vi "Drive_Cmd_Follow_Camera.vi"(9 "Forward Power":dbl, 10 "Max Turn Power":dbl, 11 "Drive Loop Cluster":T1={"Sensor Data"={"Gyro Data"={"Gyro RT FIFO"=refnum, "Gyro Current"=0.0, "Gyro Hold"=0.0}, "Encoder Data"={"Encoder RT FIFO"=refnum, "Encoder Current"=0.0, "Encoder Hold"=0.0}, "Camera Data"={"Camera RT FIFO"=refnum, "Camera Current"={" Angle"=0.0, "Valid"=FALSE}}}, "PID Update"=refnum, "RobotDriveDevRef"={"DevStatus"={"status"=FALSE, "code"=0, "source"=""}, "Motors[]"=[], "Square Inputs"=FALSE, "Max Output"=1.0}, "Drive Train"=enum."Tank Drive 2 Motor", "Valid Commands"=[], "Drive Comand Notifier"=refnum, "Command Finished?"=refnum, "Command Canceled"=refnum}) -> (0 "error out":errorcluster)   [LabVIEW 2016]
doc: "Help file written by FRC Team 836 - The RoboBees\n\nThis VI writes the \"Follow Camera\" command and power level #6 to the Drive Command RT FIFO in the Drive Loop Cluster.\n\nThe RT FIFO has to be initialized using the \"Drive_Loop_Initialize_w_Help\" VI"
uses:
  <userlib>/836-libraries/Drive/Drive_Code_V2/Drive_Code_Support/Drive_Code_Bundle.ctl
  <userlib>/836-libraries/Drive/Drive_Code_V2/Drive_Code_Support/SensorTypedefs/Sensor_Cluster.ctl
  <userlib>/836-libraries/Drive/Drive_Code_V2/Drive_Code_Support/SensorTypedefs/Camera_Cluster.ctl
  <userlib>/836-libraries/Drive/Drive_Code_V2/Drive_Code_Support/PidClusters/Drive_Code_PID_Bundle.ctl
  <vilib>/Rock Robotics/WPI/RobotDrive/WPI_RobotDriveDevRef.ctl
  <vilib>/Rock Robotics/WPI/MotorControl/WPI_MotorControlDeviceRef.ctl
  <vilib>/Rock Robotics/WPI/MotorControl/WPI_MotorControlType.ctl
  <vilib>/Rock Robotics/SystemInterfaces/DIO/FPGA_DIOPWMChannel.ctl
  <vilib>/Rock Robotics/WPI/PWM/WPI_PWMDeadband.ctl
  <userlib>/836-libraries/Drive/Drive_Code_V2/Drive_Code_Support/DriveTrains/Drive_Trains.ctl
  <userlib>/836-libraries/Drive/Drive_Code_V2/Drive_Code_Support/Command_Sends/Drive_Code_Command_Type.ctl
  <userlib>/836-libraries/Drive/Drive_Code_V2/Drive_Code_Support/Command_Sends/Drive_Code_Command_List.ctl
  <userlib>/836-libraries/Drive/Drive_Code_V2/Drive_Code_Support/Command_Sends/CommandTypeInfo/FollowCameraparam.ctl
  <vilib>/Utility/error.llb/Error Cluster From Error Code.vi
  <vilib>/ErrorRing/Error Ring.xnode
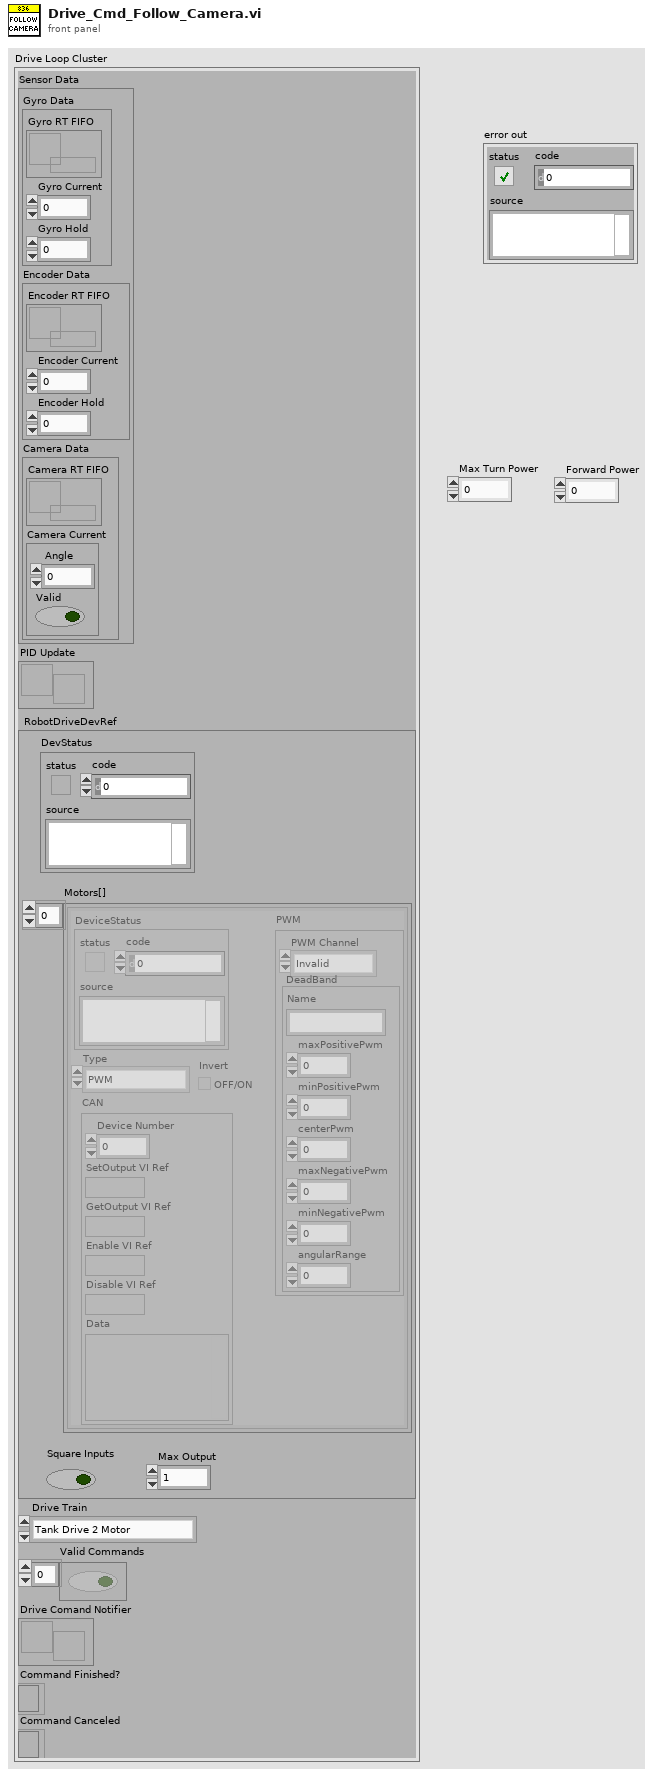
[diagram p1: front panel]
types:
  T1 = typedef "Drive_Code_Bundle.ctl" = cluster{"Sensor Data":T2, "PID Update":refnum<notifier>, "RobotDriveDevRef":T4, "Drive Train":T9, "Valid Commands":bool[], "Drive Comand Notifier":refnum<notifier>, "Command Finished?":refnum<k4>, "Command Canceled":refnum<k4>}
  T2 = typedef "Sensor_Cluster.ctl" = cluster{"Gyro Data":cluster{"Gyro RT FIFO":refnum<k33>, "Gyro Current":dbl, "Gyro Hold":dbl}, "Encoder Data":cluster{"Encoder RT FIFO":refnum<k33>, "Encoder Current":dbl, "Encoder Hold":dbl}, "Camera Data":cluster{"Camera RT FIFO":refnum<k33>, "Camera Current":T3}}
  T3 = typedef "Camera_Cluster.ctl" = cluster{" Angle":dbl, "Valid":bool}
  T4 = typedef "WPI_RobotDriveDevRef.ctl" = cluster{"DevStatus":errorcluster, "Motors[]":T5[], "Square Inputs":bool, "Max Output":dbl}
  T5 = typedef "WPI_MotorControlDeviceRef.ctl" = cluster{"DeviceStatus":errorcluster, "Type":T6, "PWM":cluster{"PWM Channel":T7, "DeadBand":T8}, "CAN":cluster{"Device Number":u8, "SetOutput VI Ref":variant, "GetOutput VI Ref":variant, "Enable VI Ref":variant, "Disable VI Ref":variant, "Data":variant}, "Invert":bool}
  T6 = typedef "WPI_MotorControlType.ctl" = enum16{"PWM", "CAN"}
  T7 = typedef "FPGA_DIOPWMChannel.ctl" = enum8{"PWM 0", "PWM 1", "PWM 2", "PWM 3", "PWM 4", "PWM 5", "PWM 6", "PWM 7", "PWM 8", "PWM 9", "PWM MXP 0", "PWM MXP 1", "PWM MXP 2", "PWM MXP 3", "PWM MXP 4", "PWM MXP 5", "PWM MXP 6", "PWM MXP 7", "PWM MXP 8", "PWM MXP 9", "Invalid"}
  T8 = typedef "WPI_PWMDeadband.ctl" = cluster{"Name":string, "maxPositivePwm":i32, "minPositivePwm":i32, "centerPwm":i32, "maxNegativePwm":i32, "minNegativePwm":i32, "angularRange":u16}
  T9 = typedef "Drive_Trains.ctl" = enum16{"Tank Drive 2 Motor", "Tank Drive 4 Motor", "Mecanum Drive", "Kiwi Drive"}
  T10 = typedef "Drive_Code_Command_List.ctl" = enum16{"Do Nothing", "Tank Drive", "Drive Continuous", "Turn", "Drive Distance", "Hold Position", "Hold Yaw", "Follow Camera", "Turn to Camera", "Approach Camera", "PID Update", "Cheesy Drive", "Update Period"}
  T11 = typedef "Drive_Code_Command_Type.ctl" = cluster{"Command":T10, "Command Params":variant}
  T12 = typedef "FollowCameraparam.ctl" = cluster{"Max Turn Power":dbl, "Forward Power":dbl}
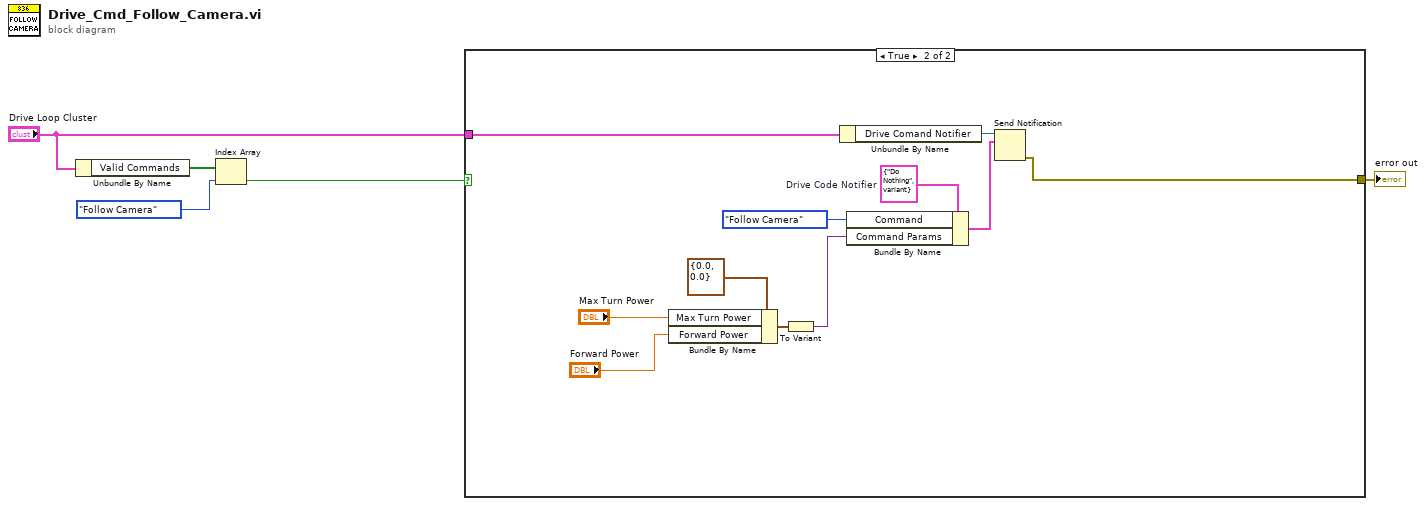
[diagram p0: block diagram]
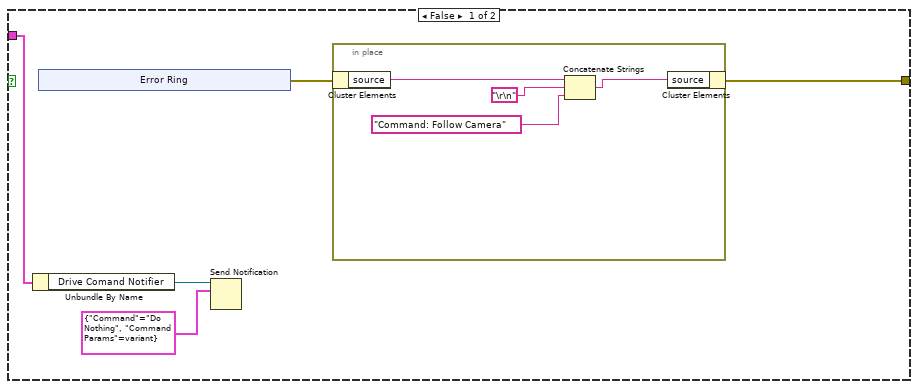
[diagram p2: hidden frame]
diagram:
  n1 = Unbundle By Name("Drive Loop Cluster") -> ("Valid Commands"=w4:bool[])
  n2 = Index Array(array=w4, index=Drive_Code_Command_List."Follow Camera" ("Command")) -> (element=w2:bool)
  n3 = case shown="True" w2 {
    tunnel: "Drive Loop Cluster" -> [w8 w22]
    tunnel: [w9 w21] -> w1
    frame False {
      n4 = Unbundle By Name(w8) -> ("Drive Comand Notifier"=w7:refnum<notifier>)
      n5 = xnode "Error Ring"() -> ("error out"=w10:errorcluster)
      n6 = Send Notification(notification=T11 {"Command"=enum."Do Nothing", "Command Params"=variant}, notifier=w7) -> ()  [unwired: 1 in, 2 out]
      n7 = in-place {
        n8 = in-place-cluster #1(w10) -> ("source"=w14:string)
        n9 = Concatenate Strings(w14, "\r\n", "Command: Follow Camera") -> (w13:string)
        n10 = in-place-cluster #1("source"=w13) -> (w9:errorcluster)
      }
    }
    frame True {
      w27 = T11 {"Command"=enum."Do Nothing", "Command Params"=variant(dbl 0.0)}  # Drive Code Notifier
      n11 = Bundle By Name(cluster=T12 {"Max Turn Power"=0.0, "Forward Power"=0.0} ("Follow Camera Param"), "Max Turn Power"="Max Turn Power", "Forward Power"="Forward Power") -> (w24:T12)
      n12 = To Variant(anything=w24) -> (Variant=w23:variant)
      n13 = Unbundle By Name(w22) -> ("Drive Comand Notifier"=w29:refnum<notifier>)
      n14 = Bundle By Name(cluster=w27, "Command"=Drive_Code_Command_List."Follow Camera", "Command Params"=w23) -> (w30:T11)
      n15 = Send Notification(notification=w30, notifier=w29) -> (error out=w21:errorcluster)  [unwired: 1 in, 1 out]
    }
  }
  "error out" <- w1
